vi "Read UI VI Ref.vi"(8 "error in (no error)":errorcluster, 11 "Subpanel Inserter in":refnum<class "Subpanel Inserter.lvclass">) -> (0 "error out":errorcluster, 2 "UI VI Ref":refnum<vi>, 3 "Subpanel Inserter out":refnum<class "Subpanel Inserter.lvclass">)   [LabVIEW 2014, in "Subpanel Insertion.lvlib" / "Subpanel Inserter.lvclass"]
uses:
  Subpanel Inserter.lvclass
  Subpanel Inserter.lvclass/Subpanel Inserter.ctl
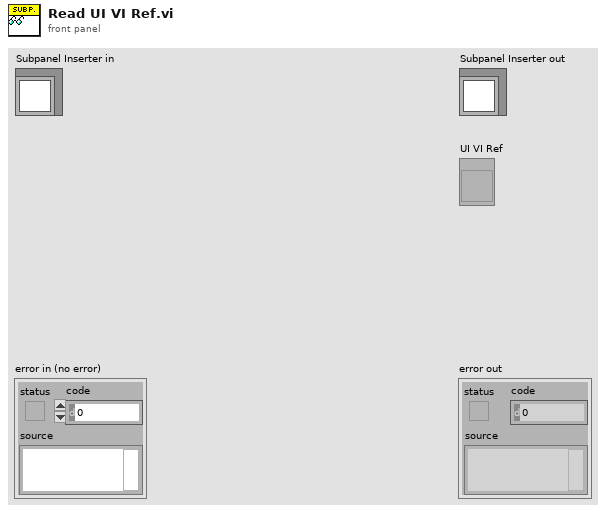
[diagram p1: front panel]
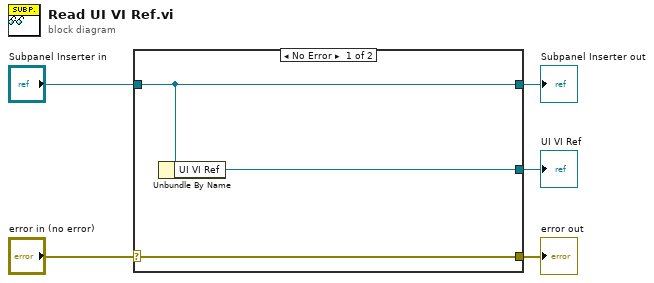
[diagram p0: block diagram]
diagram:
  n1 = case shown="No Error" "error in (no error)" {
    selector: "error in (no error)" -> [w8 w9]
    tunnel: [w8 w9] -> w4
    tunnel: [w7 w10] -> w2
    tunnel: "Subpanel Inserter in" -> [w7 w10]
    tunnel: [w6 _] -> w1
    frame No Error {
      n2 = Unbundle By Name(w7) -> ("UI VI Ref"=w6:refnum<vi>)
    }
    frame Error {
    }
  }
  "error out" <- w4
  "Subpanel Inserter out" <- w2
  "UI VI Ref" <- w1
